vi "ArmSetXZDemand.vi"(9 "SetZ":dbl, 11 "SetX":dbl) -> ()   [LabVIEW 2023]
doc: "Set XYZ demand for X,Y,Z arm globals and for ArmXYZToR-L-E, and set those outputs to ArmSetDemands\n\nInputs:\n--SetX--Double\n--SetY--Double\n--SetZ--Double"
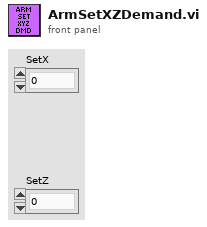
[diagram p1: front panel]
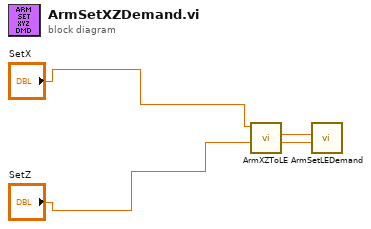
[diagram p0: block diagram]
diagram:
  n1 = call "ArmXZToLE.vi"("Z"="SetZ", "X"="SetX") -> ("Extend"=w1:dbl, "Lift"=w2:dbl)  [unwired: 8 in]
  n2 = call "ArmSetLEDemand.vi"("SetExtendPositonDemand(in)"=w1, "SetLIftPostionDemand(d)"=w2) -> ()  [unwired: 10 in]
